vi "Acquire Data.vi"(8 "error in (no error)":errorcluster, 10 "Acquire Data":bool, 11 "ARS-0220 in":refnum<class "ARS-0220.lvclass">) -> (0 "error out":errorcluster, 3 "ARS-0220 out":refnum<class "ARS-0220.lvclass">)   [LabVIEW 2021, in "Environment Chamber.lvlib" / "ARS-0220.lvclass"]
uses:
  ARS-0220.lvclass
  ARS-0220.lvclass/ARS-0220.ctl
  Support Libraries/Climatic Chamber/Climatic Chamber.lvlib
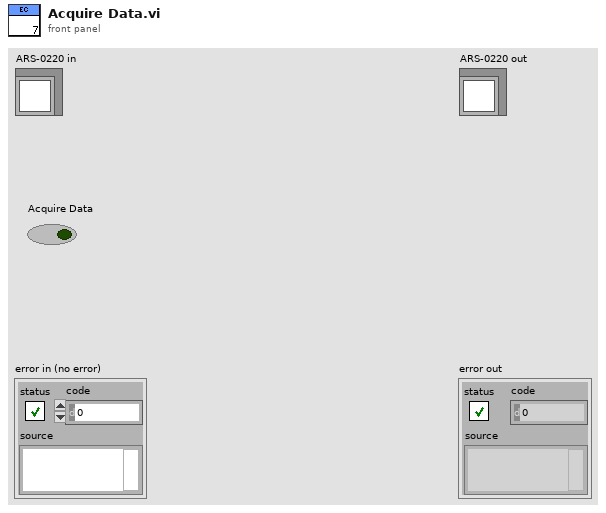
[diagram p1: front panel]
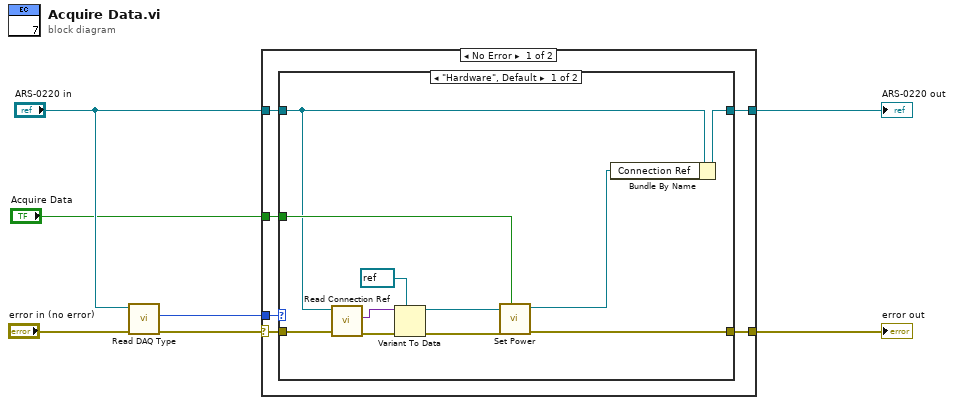
[diagram p0: block diagram]
diagram:
  n1 = call "Read DAQ Type.vi"("error in (no error)"="error in (no error)", "ARS-0220 in"="ARS-0220 in") -> ("error out"=w6:errorcluster, "DAQ Type"=w4:enum16{"Hardware", "Simulation"})  [unwired: 7 in, 1 out]
  n2 = case shown="No Error" w6 {
    selector: w6 -> [w10 w27]
    tunnel: "ARS-0220 in" -> [w11 w28]
    tunnel: w4 -> [w13 _]
    tunnel: "Acquire Data" -> [w12 _]
    tunnel: [w9 w27] -> w2
    tunnel: [w8 w28] -> w1
    frame No Error {
      n3 = case shown="\"Hardware\", Default" w13 {
        tunnel: w12 -> [w20 _]
        tunnel: w11 -> [w16 w26]
        tunnel: w10 -> [w24 w25]
        tunnel: [w17 w25] -> w9
        tunnel: [w15 w26] -> w8
        frame "Hardware", Default {
          n4 = call "Read Connection Ref.vi"("error in (no error)"=w24, "ARS-0220 in"=w16) -> ("error out"=w23:errorcluster, "Connection Ref"=w22:variant)  [unwired: 7 in, 1 out]
          n5 = Variant To Data(error in=w23, type=refnum<visa-resource-name> refnum ("VISA resource name"), Variant=w22) -> (data=w18:refnum<visa-resource-name>, error out=w21:errorcluster)
          n6 = call "Set Power.vi"("Power (On/Off)"=w20, "error in (no error)"=w21, "VISA resource name"=w18) -> ("error out"=w17:errorcluster, "VISA resource name out"=w14:refnum<visa-resource-name>)  [unwired: 7 in]
          n7 = Bundle By Name(cluster=w16, "Connection Ref"=w14) -> (w15:refnum<class "ARS-0220.lvclass">)
        }
        frame "Simulation" {
        }
      }
    }
    frame Error {
    }
  }
  "error out" <- w2
  "ARS-0220 out" <- w1
